vi "sub_Init_MFSK_At_RX.vi"(6 "PN sequence order (9)":i32=9, 7 "synchronization parameters":T3={"expected sync location (symbols)"=-1, "sync sequence"=[], "sync location uncertainty (symbols)"=0, "sync indent (symbols)"=0} {"sync sequence" format="%.2f"}, 8 "filter parameters":T4={"Alpha"=0.5, "Filter Length"=6, "TX Filter"=enum."Root Raised Cos"} {"Alpha" format="%.2f"}, 9 "Sync Bits":i32=20, 10 "FSK Parameters":T1) -> (1 "FSK Init Parameters":T2)   [LabVIEW 2015]
uses:
  <vilib>/addons/Modulation/Digital/General/MT Generate Bits (Galois, PN Order).vi
  <vilib>/addons/Modulation/Digital/Support/Common/Validators/mod_Generate Bits Validate.vi
  <vilib>/addons/Modulation/Analog/support/mod_Set Error Source.vi
  <vilib>/addons/Modulation/Digital/General/subVIs/mod_Generate Bits PN Sequence.vi
  <vilib>/addons/Modulation/Digital/General/MT Generate FSK System Parameters(M).vi
  <vilib>/addons/Modulation/Digital/Support/Common/Validators/mod_Generate Filter Coefficients Validate.vi
  <vilib>/addons/Modulation/Digital/General/subVIs/mod_Generate Filter Coefficients.vi
  <vilib>/addons/Modulation/Digital/General/MT Map Bits to FSK Symbols.vi
  <vilib>/addons/Modulation/niDMT.lvlib
panel:
  in  "error in (no error)":errorcluster
  out "error out":errorcluster
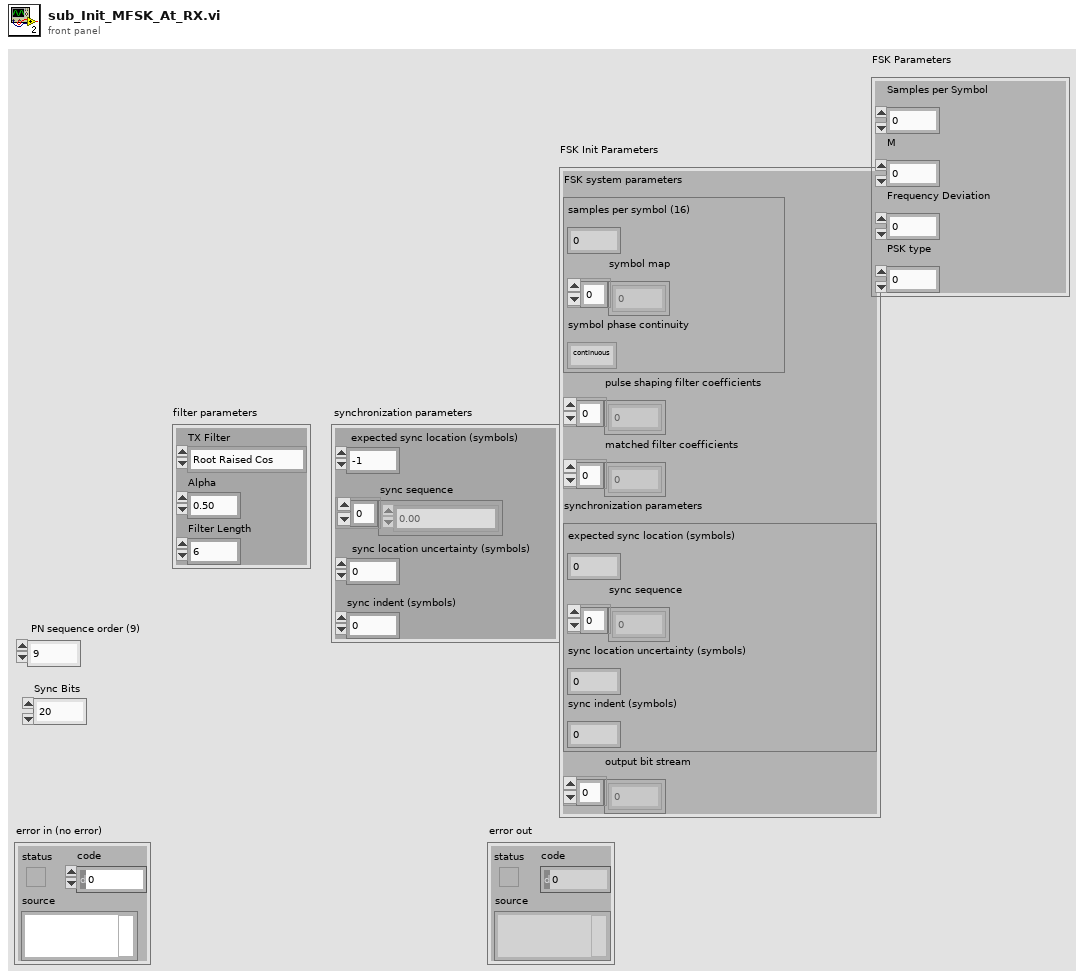
[diagram p1: front panel]
types:
  T1 = cluster{"Samples per Symbol":i32, "M":i32, "Frequency Deviation":dbl, "PSK type":u16}
  T2 = cluster{"FSK system parameters":cluster{"samples per symbol (16)":i32, "symbol map":dbl[], "symbol phase continuity":enum16{"continuous", "discontinuous"}}, "pulse shaping filter coefficients":dbl[], "matched filter coefficients":dbl[], "synchronization parameters":cluster{"expected sync location (symbols)":i32, "sync sequence":cdb[], "sync location uncertainty (symbols)":i32, "sync indent (symbols)":i32}, "output bit stream":i8[]}
  T3 = cluster{"expected sync location (symbols)":i32, "sync sequence":cdb[], "sync location uncertainty (symbols)":i32, "sync indent (symbols)":i32}
  T4 = cluster{"Alpha":dbl, "Filter Length":i32, "TX Filter":enum16{"none", "Raised Cosine", "Root Raised Cos", "Gaussian"}}
  T5 = enum16{"FSK", "PSK", "QAM", "MSK", "PAM", "ASK", "CPM"}
  T6 = enum16{"none", "Raised Cosine", "Root Raised Cos", "Gaussian"}
  T7 = cluster{"samples per symbol (16)":i32, "symbol map":dbl[], "symbol phase continuity":enum16{"continuous", "discontinuous"}}
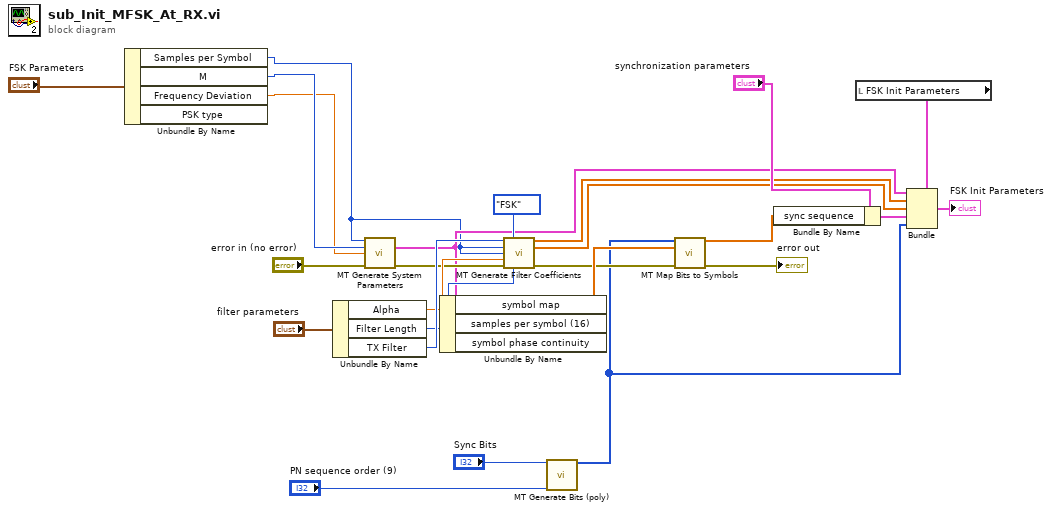
[diagram p0: block diagram]
diagram:
  n1 = Unbundle By Name("FSK Parameters") -> ("Samples per Symbol"=w3:i32, "M"=w2:i32, "Frequency Deviation"=w1:dbl)  [unwired: 1 out]
  n2 = Unbundle By Name("filter parameters") -> ("Alpha"=w20:dbl, "Filter Length"=w21:i32, "TX Filter"=w22:T6)
  n3 = call-poly <vilib>:"MT Generate System Parameters.vi"("samples per symbol (16)"=w3, "M-FSK (2)"=w2, "FSK deviation (Hz)"=w1, "error in (no error)"="error in (no error)") -> ("FSK system parameters"=w7:T7, "error out"=w18:errorcluster)  [unwired: 9 in, 1 out]
  n4 = Unbundle By Name(w7) -> ("symbol map"=w23:dbl[])  [unwired: 2 out]
  n5 = call <vilib>:"MT Generate Filter Coefficients.vi"("pulse shaping filter (none)"=w22, "modulation type"=T5."FSK", "pulse shaping samples per symbol (16)"=w3, "matched samples per symbol (16)"=w3, "filter parameter"=w20, "error in (no error)"=w18, "filter length (symbols)"=w21) -> ("pulse shaping filter coefficients"=w11:dbl[], "matched filter coefficients"=w15:dbl[], "error out"=w14:errorcluster)  [unwired: 6 in]
  n6 = call-poly <vilib>:"MT Generate Bits (poly).vi"("total bits (128)"="Sync Bits", "PN sequence order (9)"="PN sequence order (9)") -> ("output bit stream"=w10:i8[])  [unwired: 11 in, 2 out]
  n7 = call-poly <vilib>:"MT Map Bits to Symbols.vi"("input bit stream"=w10, "symbol map"=w23, "error in (no error)"=w14) -> ("symbols"=w24:dbl[], "error out"=→"error out":errorcluster)  [unwired: 11 in]
  n8 = Bundle By Name(cluster="synchronization parameters", "sync sequence"=w24) -> (w16:T3)
  n9 = local read "FSK Init Parameters"() -> (w5:T2)
  n10 = Bundle(cluster=w5, "FSK system parameters"=w7, "pulse shaping filter coefficients"=w11, "matched filter coefficients"=w15, "synchronization parameters"=w16, "output bit stream"=w10) -> (→"FSK Init Parameters":T2)
